vi "fgv_TM-arr.vi"(7 "cmd":T1, 10 "arr limit":i32=200, 11 "TM":cluster{"Y(E)":dbl, "X(N)":dbl}) -> (3 "TM array":cluster{"Y(E)":dbl, "X(N)":dbl}[](array[cluster]))   [LabVIEW 2019]
uses:
  Ctrl/cmd_ini-add-read.ctl
  Ctrl/cmd_common.ctl
panel:
  out "Points size":i32
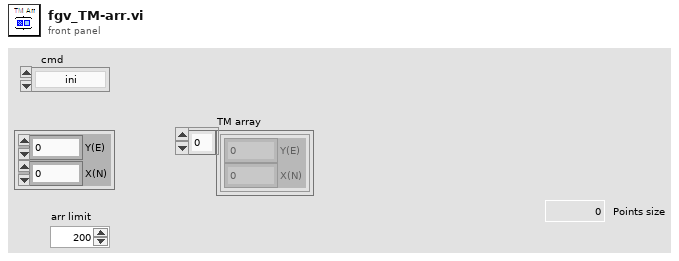
[diagram p1: front panel]
types:
  T1 = typedef "cmd_ini-add-read.ctl" = enum16{"ini", "add", "read"}
  T2 = typedef "cmd_common.ctl" = enum16{"read", "write"}
  T3 = typedef "GNSS-Ntrip config.ctl" = cluster{"Current NtripClient Account":cluster{"id":string, "pwd":string, "ref pt":string, "address":string, "port ":u16}, "Mount points":u16, "Ref r size":dbl, "TMarr limit":i32, "Sel NMEA type":enum16{"$GPGSV", "$GLGSV", "$GPGGA", "$GAGSV", "$GBGSV", "$GNGLL", "$GNGGA", "$GNGSA", "$GNRMC", "$GNVTG"}, "Local Time offset":u32, "Write delay ms":u32, "GNSS Serial delay":u32, "Send Serial delay":u32, "Ntrip accounts":cluster{"id":string, "pwd":string, "ref pt":string, "address":string, "port ":u16}[], "Send Serial config":cluster{"NMEA out port":refnum<visa-resource-name>, "baud rate":u32}, "Mount point arr":string[]}
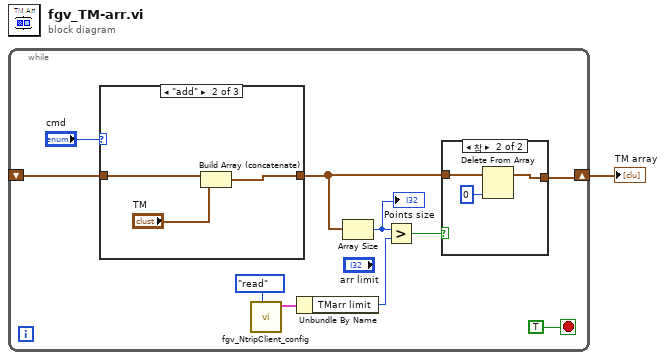
[diagram p0: block diagram]
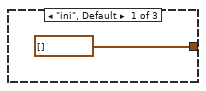
[diagram p3: hidden frame]
diagram:
  n1 = while {
    shift-right: [w5] -> w1
    shift-left: _ -> [w9]
    stop <- TRUE stop-if-true
    n2 = case shown="\"add\"" "cmd" {
      tunnel: [cluster{"Y(E)":dbl, "X(N)":dbl}[] [] w19 w20] -> w6
      tunnel: w9 -> [_ w18 w20]
      frame "ini", Default {
      }
      frame "add" {
        n3 = Build Array (concatenate)(w18, "TM") -> (w19:cluster{"Y(E)":dbl, "X(N)":dbl}[])
      }
      frame "read" {
      }
    }
    n4 = call "fgv_NtripClient_config.vi"("cmd"=cmd_common."read") -> ("config val out"=w3:T3)  [unwired: 10 in]
    n5 = Unbundle By Name(w3) -> ("TMarr limit"=w2:i32)
    n6 = Array Size(array=w6) -> (size(s)=w8:i32)
    "Points size" <- w8
    n7 = Greater?(x=w8, y=w2) -> (0:w7:bool)
    n8 = case shown="참" w7 {
      tunnel: w6 -> [w12 w14]
      tunnel: [w12 w13] -> w5
      frame False {
      }
      frame True {
        n9 = Delete From Array(array=w14, index=0) -> (array with subset deleted=w13:cluster{"Y(E)":dbl, "X(N)":dbl}[])  [unwired: 1 in, 1 out]
      }
    }
  }
  "TM array" <- w1
